vi "XNet Type to Tag Bus Type.vi"(10 "Data Type":u32(ring) items=["Signed", "Unsigned", "IEEE Float"], 11 "NumBits":u32) -> (3 "data type":T1)   [LabVIEW 2013, in "J1939.lvlib"]
uses:
  J1939.lvlib
  <vilib>/NI/Tag Bus/tag/Data Type.ctl
  <vilib>/NI/Tag Bus/tag/tag descriptor.lvclass
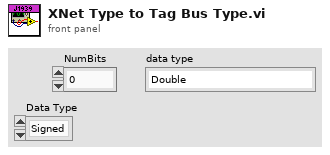
[diagram p1: front panel]
types:
  T1 = typedef "tag bus.lvlib/tag descriptor.lvclass/Data Type.ctl" = enum16{"Double", "Single", "I64", "I32", "I16", "I8", "U64", "U32", "U16", "U8", "Boolean", "String", "Array of Double", "Array of Single", "Array of I64", "Array of I32", "Array of I16", "Array of I8", "Array of U64", "Array of U32", "Array of U16", "Array of U8", "Array of Boolean", "Array of String"}
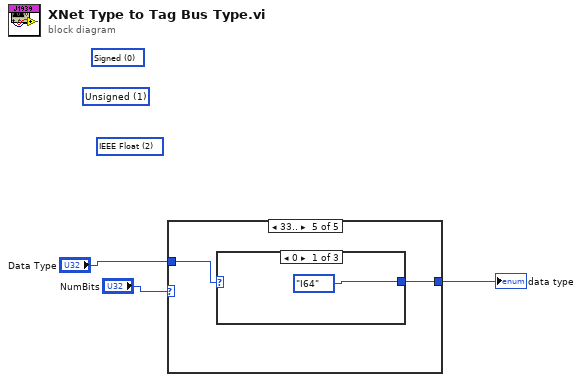
[diagram p0: block diagram]
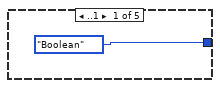
[diagram p2: hidden frame]
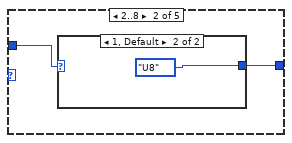
[diagram p3: hidden frame]
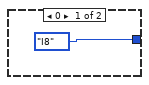
[diagram p4: hidden frame]
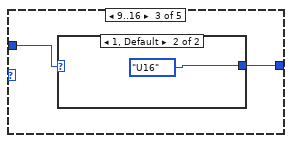
[diagram p5: hidden frame]
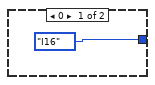
[diagram p6: hidden frame]
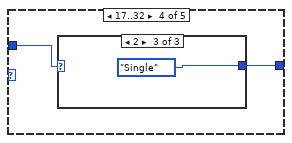
[diagram p7: hidden frame]
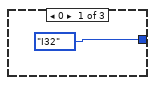
[diagram p8: hidden frame]
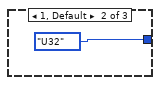
[diagram p9: hidden frame]
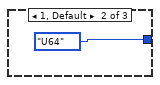
[diagram p10: hidden frame]
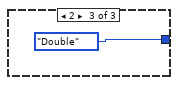
[diagram p11: hidden frame]
diagram:
  (unwired) u32 2 items=["Signed", "Unsigned", "IEEE Float"] ("Data Type")
  (unwired) u32 1 items=["Signed", "Unsigned", "IEEE Float"] ("Data Type")
  (unwired) u32 0 items=["Signed", "Unsigned", "IEEE Float"] ("Data Type")
  n1 = case shown="33.." "NumBits" {
    tunnel: [Data_Type."Boolean" ("data type") w6 w10 w14 w19] -> w2
    tunnel: "Data Type" -> [_ w5 w9 w13 w18]
    frame ..1 {
    }
    frame 2..8 {
      n2 = case shown="1, Default" w5 {
        tunnel: [Data_Type."I8" ("data type") Data_Type."U8" ("data type")] -> w6
        frame 0 {
        }
        frame 1, Default {
        }
      }
    }
    frame 9..16 {
      n3 = case shown="1, Default" w9 {
        tunnel: [Data_Type."I16" ("data type") Data_Type."U16" ("data type")] -> w10
        frame 0 {
        }
        frame 1, Default {
        }
      }
    }
    frame 17..32 {
      n4 = case shown="2" w13 {
        tunnel: [Data_Type."I32" ("data type") Data_Type."U32" ("data type") Data_Type."Single" ("data type")] -> w14
        frame 0 {
        }
        frame 1, Default {
        }
        frame 2 {
        }
      }
    }
    frame 33.. {
      n5 = case shown="0" w18 {
        tunnel: [Data_Type."I64" ("data type") Data_Type."U64" ("data type") Data_Type."Double" ("data type")] -> w19
        frame 0 {
        }
        frame 1, Default {
        }
        frame 2 {
        }
      }
    }
  }
  "data type" <- w2
